vi "SC_schleife_mischer.vi"() -> ()   [LabVIEW 2019]
uses:
  Global/Global Variables/global.vi
  Global/Global Variables/Data_Display_global.vi
  Instrument_Setup.vi
  <vilib>/Analysis/NI_AALBase.lvlib
  <vilib>/Analysis/NI_AALPro.lvlib
panel:
  out "Numeric":dbl format="%#_13g"
  out "Array":dbl[](array[numeric])
  out "Numeric 5":dbl format="%#_13g"
  out "Numeric 4":dbl format="%#_13g"
  out "XY Graph 2":T1(graph)
  out "XY Graph":T1(graph)
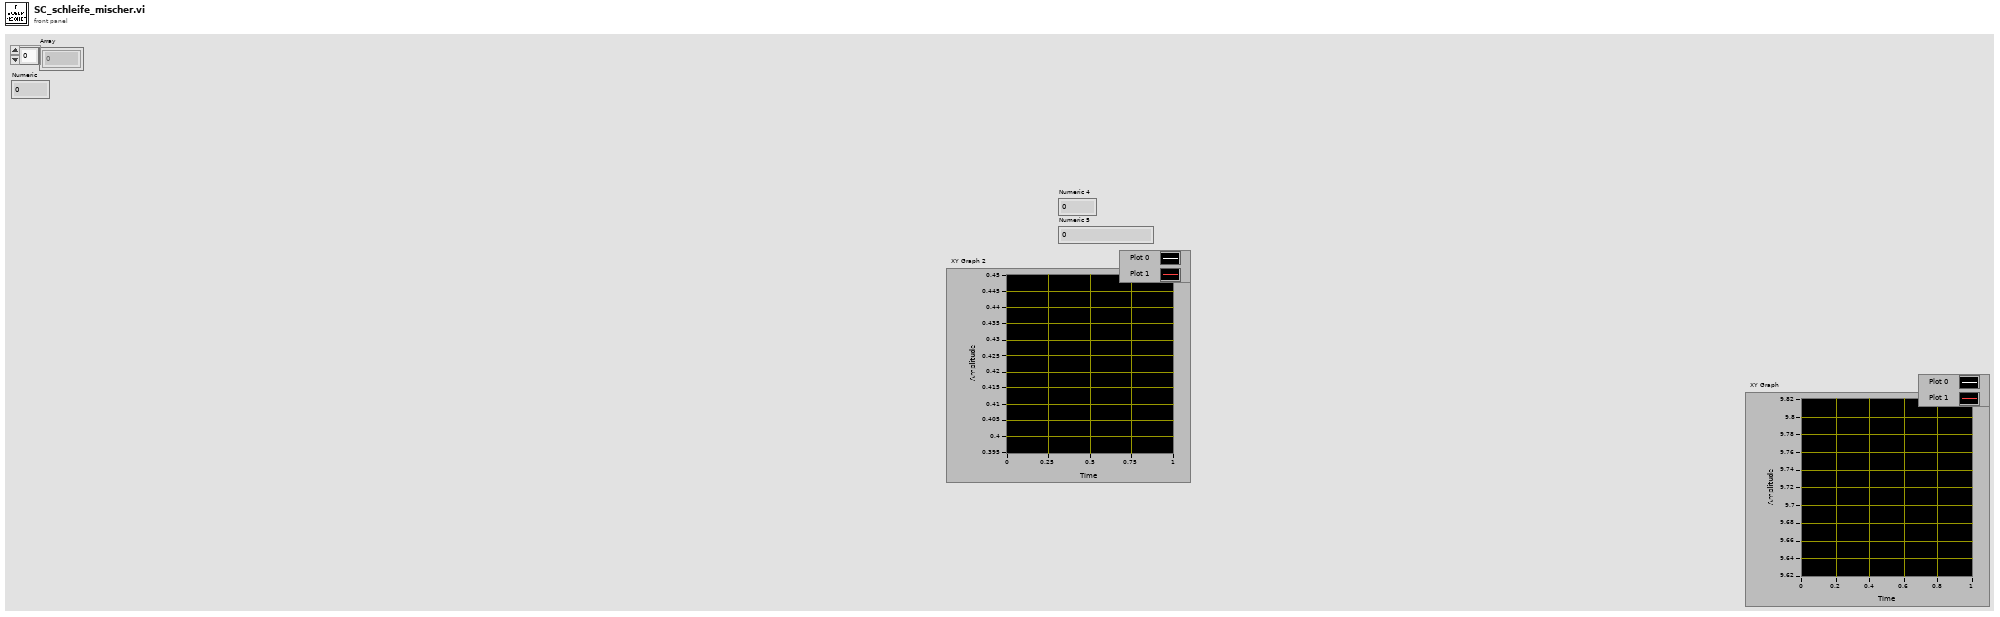
[diagram p1: front panel]
types:
  T1 = cluster{"Plot1":dbl[], "Best Linear Fit":dbl[]}[]
  T2 = typedef "LS372-Cluster.ctl" = cluster{"Activate Tsweep":bool, "Setpoint - Manual":dbl, "Rate (K/min)":dbl, "Update Lakeshores":bool, "Still Heater":bool, "Still Power (mW)":dbl, "Manual Heater":bool, "Manual Heater  (mW) ":dbl, "Heater Range":dbl, "P (Gain)":dbl, "I (Reset)":dbl, "D (Rate)":dbl, "Heater Power (mW)":dbl, "MC Thermometer":u16, "MC Temperature":dbl, "LS372-T1":dbl, "LS372 -T2":dbl, "LS372-R1 ":dbl, "LS372-R2":dbl, "LS372-T3":dbl, "LS372-T4":dbl, "LS372-R3 ":dbl, "LS372-R4 \n\n\n\n":dbl, "LS372-T5":dbl, "LS372-T6":dbl, "LS372-R5":dbl, "LS372-R6 ":dbl, "Still Power ist":dbl, "Set Temperatur Sweep main":bool, "Setpoint ist":dbl, "Disable Heater":bool}
  T3 = typedef "Ls372-Control.ctl" = cluster{"Activate Tsweep":bool, "Setpoint - Manual":dbl, "Rate (K/min)":dbl, "Update Lakeshores":bool, "Still Heater":bool, "Still Power (mW)":dbl, "Manual Heater":bool, "Manual Heater  (mW) ":dbl, "MC Thermometer":u16, "Set Temperature Sweeep main":bool, "Disable Heater":bool}
  T4 = typedef "LS350-cluster.ctl" = cluster{"Setpoint":dbl, "Heater Output":dbl, "Setpoint control":dbl, "Enable Setpoint":bool, "LS350 T1":dbl, "LS350 T2":dbl, "LS350 T3":dbl, "LS350 T4":dbl, "LS350 R1":dbl, "LS350 R2":dbl, "LS350 R3":dbl, "LS350 R4":dbl}
  T5 = cluster{"Plot 1":dbl[], "Best Linear Fit":dbl[]}[]
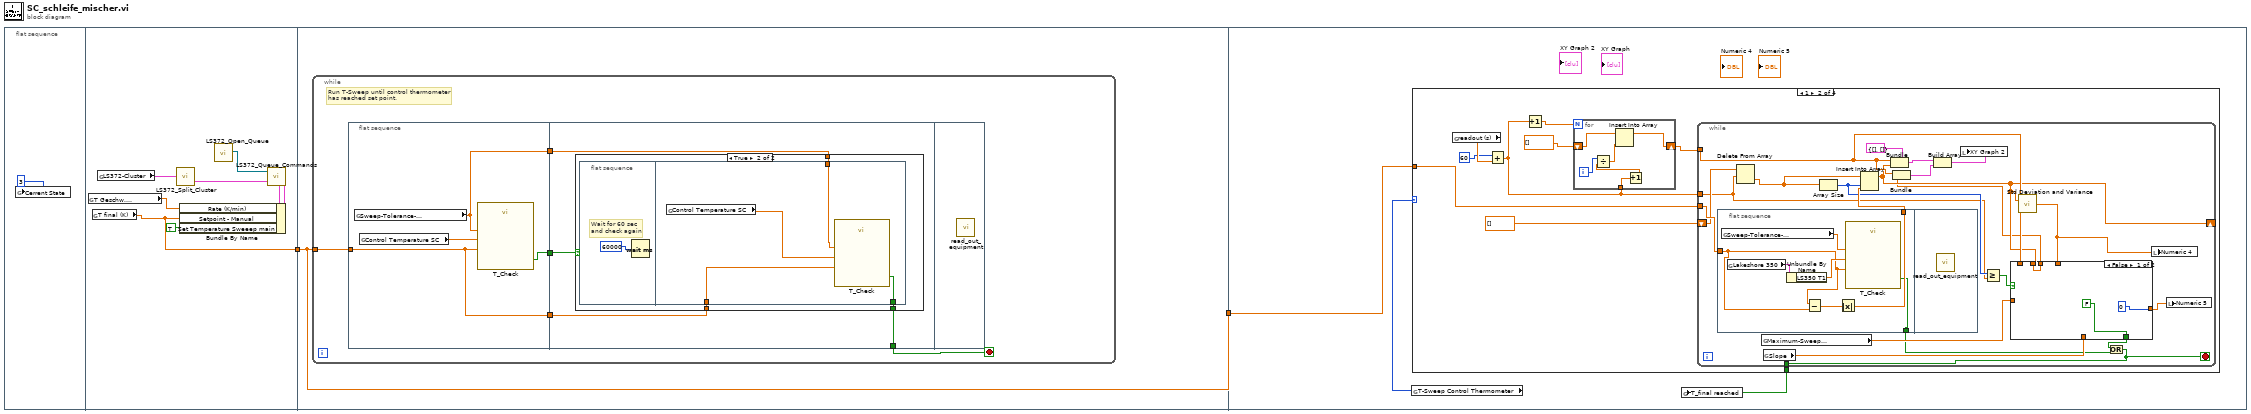
[diagram p0: block diagram]
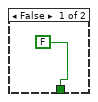
[diagram p2: hidden frame]
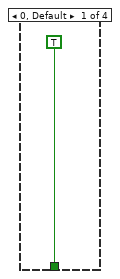
[diagram p3: hidden frame]
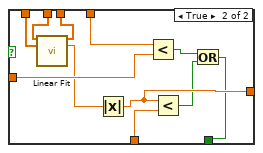
[diagram p4: hidden frame]
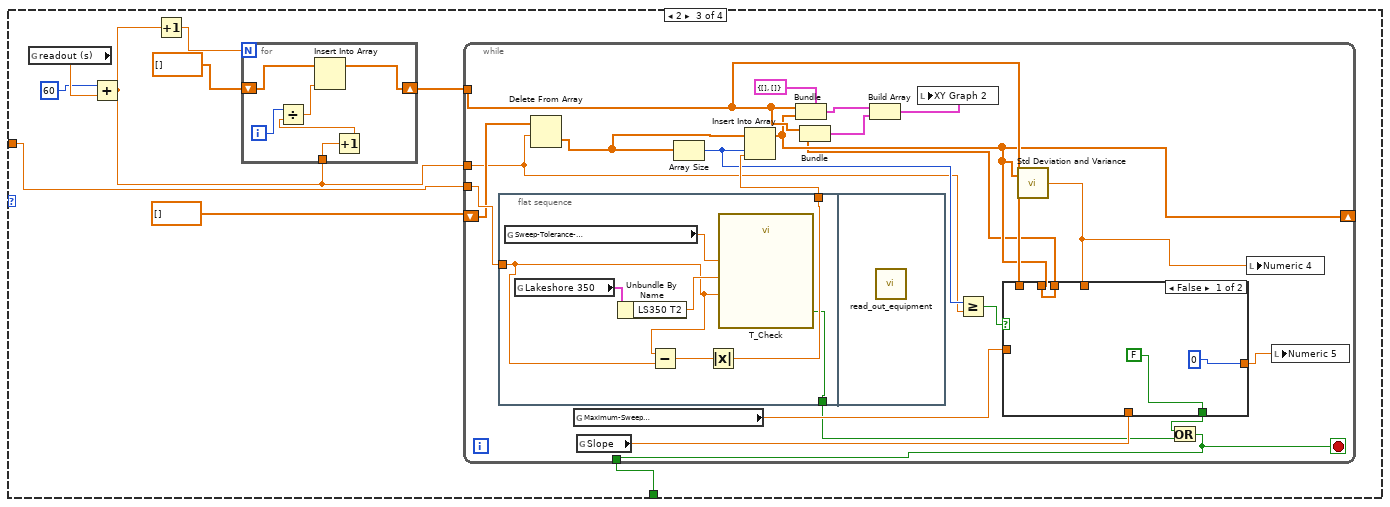
[diagram p5: hidden frame]
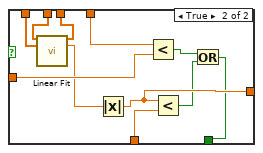
[diagram p6: hidden frame]
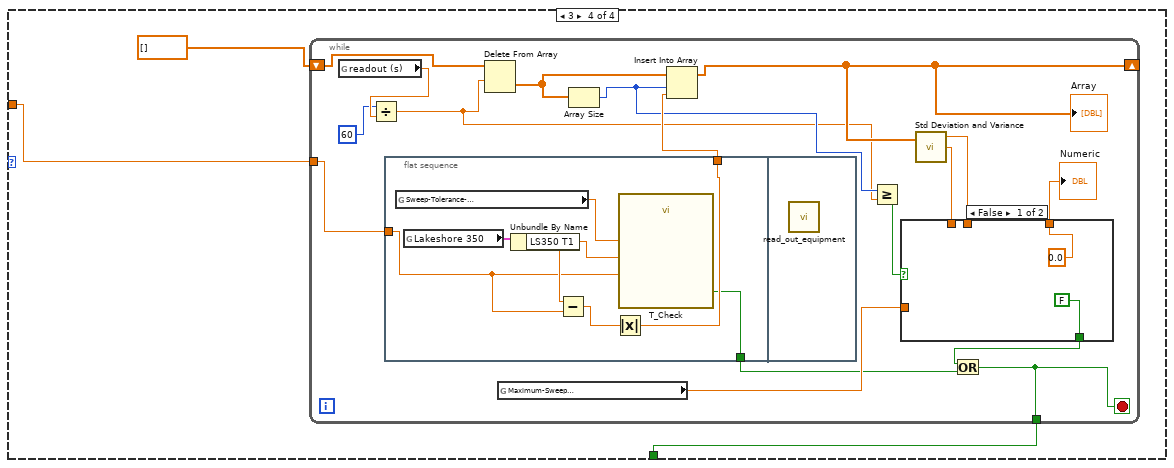
[diagram p7: hidden frame]
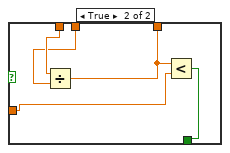
[diagram p8: hidden frame]
diagram:
  n1 = flat-sequence {
    tunnel: [w4] -> w2
    tunnel: w2 -> [w11]
    tunnel: [w11] -> w1
    tunnel: w1 -> [w35]
    frame #0 {
      n2 = global write "global.vi" "Cerrent State"(3) -> ()
    }
    frame #1 {
      n3 = global read "global.vi" "T Geschw. \n(K/min)"() -> (w7:dbl)
      n4 = global read "global.vi" "T final (K)"() -> (w4:dbl)
      n5 = global read "Data_Display_global.vi" "LS372-Cluster"() -> (w10:T2)
      n6 = call "LS372_Split_Cluster.vi"("LS372-Cluster"=w10) -> ("LS372-Control"=w9:T3)  [unwired: 1 out]
      n7 = Bundle By Name(cluster=w9, "Rate (K/min)"=w7, "Setpoint - Manual"=w4, "Set Temperature Sweeep main"=TRUE) -> (w5:T3)
      n8 = call "LS372_Open_Queue.vi"() -> ("queue out"=w6:refnum<queue>)  [unwired: 10 in, 1 out]
      n9 = call "LS372_Queue_Commands.vi"("LS372-Control"=w5, "Queue"=w6) -> ()  [unwired: 1 in, 1 out]
    }
    frame #2 {
      n10 = while {
        tunnel: w11 -> [w16]
        stop <- w12 stop-if-true
        # "Run T-Sweep until control thermometer\nhas reached set point."
        n11 = flat-sequence {
          tunnel: w16 -> [w18]
          tunnel: [w19] -> w15
          tunnel: [w18] -> w14
          tunnel: [w17] -> w13
          tunnel: w15 -> [w24]
          tunnel: w14 -> [w23]
          tunnel: w13 -> [w22]
          tunnel: [w21] -> w12
          frame #0 {
            n12 = global read "Instrument_Setup.vi" "Sweep-Tolerance-\nTemperature"() -> (w19:dbl)
            n13 = global read "Data_Display_global.vi" "Control Temperature SC"() -> (w20:dbl)
            n14 = call "T_Check.vi"("Sweep\nTolerance %"=w19, "T_target (K)"=w18, "T_in"=w20) -> ("= T target"=w17:bool)
          }
          frame #1 {
            n15 = case shown="True" w22 {
              tunnel: w23 -> [_ w28]
              tunnel: w24 -> [_ w27]
              tunnel: [FALSE w26] -> w21
              frame False {
              }
              frame True {
                n16 = flat-sequence {
                  tunnel: w28 -> [w33]
                  tunnel: w27 -> [w32]
                  tunnel: [w31] -> w26
                  frame #0 {
                    # "Wait for 60 sec\nand check again"
                    n17 = Wait (ms)(milliseconds to wait=60000) -> ()  [unwired: 1 out]
                  }
                  frame #1 {
                    n18 = global read "Data_Display_global.vi" "Control Temperature SC"() -> (w30:dbl)
                    n19 = call "T_Check.vi"("Sweep\nTolerance %"=w32, "T_target (K)"=w33, "T_in"=w30) -> ("= T target"=w31:bool)
                  }
                }
              }
            }
          }
          frame #2 {
            n20 = call "read_out_equipment.vi"() -> ()  [unwired: 1 in]
          }
        }
      }
    }
    frame #3 {
      n21 = global read "Instrument_Setup.vi" "T-Sweep Control Thermometer"() -> (w36:u16)
      n22 = case shown="1" w36 {
        tunnel: w35 -> [_ w41 w96 w154]
        tunnel: [TRUE w38 w103 w152] -> w34
        frame 0, Default {
        }
        frame 1 {
          n23 = global read "Instrument_Setup.vi" "readout (s)"() -> (w46:dbl)
          n24 = Add(x=60, y=w46) -> (x+y=w39:dbl)
          n25 = Increment(x=w39) -> (x+1=w44:dbl)
          n26 = for {
            N: w44 -> [_]
            shift-right: [w91] -> w40
            shift-left: dbl[] [] -> [w93]
            tunnel: w39 -> [w90]
            i -> [w94]
            n27 = Increment(x=w90) -> (x+1=w89:dbl)
            n28 = Divide(x=w94, y=w89) -> (x/y=w92:dbl)
            n29 = Insert Into Array(array=w93, new element=w92) -> (w91:dbl[])  [unwired: 1 in]
          }
          n30 = while {
            shift-right: [w56] -> _
            shift-left: dbl[] [] -> [w66]
            tunnel: w41 -> [w67]
            tunnel: w40 -> [w59]
            tunnel: w39 -> [w57]
            tunnel: [w47] -> w38
            stop <- w47 stop-if-true
            n31 = flat-sequence {
              tunnel: w67 -> [w85]
              tunnel: [w83] -> w63
              tunnel: [w82] -> w49
              frame #0 {
                n32 = global read "Instrument_Setup.vi" "Sweep-Tolerance-\nTemperature"() -> (w88:dbl)
                n33 = global read "Data_Display_global.vi" "Lakeshore 350"() -> (w87:T4)
                n34 = Unbundle By Name(w87) -> ("LS350 T1"=w86:dbl)
                n35 = Subtract(x=w85, y=w85) -> (x-y=w84:dbl)
                n36 = Absolute Value(x=w84) -> (abs(x)=w83:dbl)
                n37 = call "T_Check.vi"("Sweep\nTolerance %"=w88, "T_target (K)"=w85, "T_in"=w86) -> ("= T target"=w82:bool)
              }
              frame #1 {
                n38 = call "read_out_equipment.vi"() -> ()  [unwired: 1 in]
              }
            }
            n39 = Delete From Array(array=w66, length=w57) -> (deleted portion=w64:dbl[])  [unwired: 1 in, 1 out]
            n40 = global read "Instrument_Setup.vi" "Maximum-Sweep\nSettle %/min"() -> (w52:dbl)
            n41 = global read "Instrument_Setup.vi" "Slope"() -> (w51:dbl)
            n42 = Array Size(array=w64) -> (size(s)=w58:i32)
            n43 = Insert Into Array(array=w64, index=w58, new element=w63) -> (w56:dbl[])
            n44 = Bundle(cluster=cluster{"Plot 1":dbl[], "Plot 2":dbl[]} {"Plot 1"=[], "Plot 2"=[]}, "Plot 1"=w59, "Plot 2"=w56) -> (w62:cluster{"Plot 1":dbl[], "Plot 2":dbl[]})
            n45 = Greater Or Equal?(x=w58, y=w57) -> (x >= y?=w53:bool)
            n46 = call <vilib>:"Std Deviation and Variance.vi"("X"=w56) -> ("standard deviation"=w55:dbl)  [unwired: 1 in, 2 out]
            n47 = case shown="False" w53 {
              tunnel: w56 -> [w68 w80]
              tunnel: w59 -> [_ w81]
              tunnel: w55 -> [_ w78]
              tunnel: [w68 w79] -> w54
              tunnel: w52 -> [_ w77]
              tunnel: w51 -> [_ w75]
              tunnel: [0 w74] -> w50
              tunnel: [FALSE w71] -> w48
              frame False {
              }
              frame True {
                n48 = call <vilib>:"Linear Fit.vi"("Y"=w80, "X"=w81) -> ("Best Linear Fit"=w79:dbl[], "slope"=w76:dbl)  [unwired: 9 in, 3 out]
                n49 = Absolute Value(x=w76) -> (abs(x)=w74:dbl)
                n50 = Less?(x=w78, y=w77) -> (x < y?=w73:bool)
                n51 = Less?(x=w74, y=w75) -> (x < y?=w72:bool)
                n52 = Or(x=w73, y=w72) -> (x .or. y?=w71:bool)
              }
            }
            n53 = Bundle(w59, "Best Linear Fit"=w54) -> (w61:cluster{dbl[], "Best Linear Fit":dbl[]})  [unwired: 1 in]
            n54 = Build Array(w62, w61) -> (w60:T5)
            n55 = local write "XY Graph 2"(w60) -> ()
            n56 = Or(x=w48, y=w49) -> (x .or. y?=w47:bool)
            n57 = local write "Numeric 4"(w55) -> ()
            n58 = local write "Numeric 5"(w50) -> ()
          }
        }
        frame 2 {
          n59 = global read "Instrument_Setup.vi" "readout (s)"() -> (w102:dbl)
          n60 = Add(x=60, y=w102) -> (x+y=w97:dbl)
          n61 = Increment(x=w97) -> (x+1=w100:dbl)
          n62 = for {
            N: w100 -> [_]
            shift-right: [w106] -> w98
            shift-left: dbl[] [] -> [w108]
            tunnel: w97 -> [w105]
            i -> [w109]
            n63 = Increment(x=w105) -> (x+1=w104:dbl)
            n64 = Divide(x=w109, y=w104) -> (x/y=w107:dbl)
            n65 = Insert Into Array(array=w108, new element=w107) -> (w106:dbl[])  [unwired: 1 in]
          }
          n66 = while {
            shift-right: [w119] -> _
            shift-left: dbl[] [] -> [w129]
            tunnel: w96 -> [w130]
            tunnel: w98 -> [w122]
            tunnel: w97 -> [w120]
            tunnel: [w110] -> w103
            stop <- w110 stop-if-true
            n67 = flat-sequence {
              tunnel: w130 -> [w148]
              tunnel: [w146] -> w126
              tunnel: [w145] -> w112
              frame #0 {
                n68 = global read "Instrument_Setup.vi" "Sweep-Tolerance-\nTemperature"() -> (w151:dbl)
                n69 = global read "Data_Display_global.vi" "Lakeshore 350"() -> (w150:T4)
                n70 = Unbundle By Name(w150) -> ("LS350 T2"=w149:dbl)
                n71 = Subtract(x=w148, y=w148) -> (x-y=w147:dbl)
                n72 = Absolute Value(x=w147) -> (abs(x)=w146:dbl)
                n73 = call "T_Check.vi"("Sweep\nTolerance %"=w151, "T_target (K)"=w148, "T_in"=w149) -> ("= T target"=w145:bool)
              }
              frame #1 {
                n74 = call "read_out_equipment.vi"() -> ()  [unwired: 1 in]
              }
            }
            n75 = Delete From Array(array=w129, length=w120) -> (deleted portion=w127:dbl[])  [unwired: 1 in, 1 out]
            n76 = global read "Instrument_Setup.vi" "Maximum-Sweep\nSettle %/min"() -> (w115:dbl)
            n77 = global read "Instrument_Setup.vi" "Slope"() -> (w114:dbl)
            n78 = Array Size(array=w127) -> (size(s)=w121:i32)
            n79 = Insert Into Array(array=w127, index=w121, new element=w126) -> (w119:dbl[])
            n80 = Bundle(cluster=cluster{"Plot 1":dbl[], "Plot 2":dbl[]} {"Plot 1"=[], "Plot 2"=[]}, "Plot 1"=w122, "Plot 2"=w119) -> (w125:cluster{"Plot 1":dbl[], "Plot 2":dbl[]})
            n81 = Greater Or Equal?(x=w121, y=w120) -> (x >= y?=w116:bool)
            n82 = call <vilib>:"Std Deviation and Variance.vi"("X"=w119) -> ("standard deviation"=w118:dbl)  [unwired: 1 in, 2 out]
            n83 = case shown="False" w116 {
              tunnel: w119 -> [w131 w143]
              tunnel: w122 -> [_ w144]
              tunnel: w118 -> [_ w141]
              tunnel: [w131 w142] -> w117
              tunnel: w115 -> [_ w140]
              tunnel: w114 -> [_ w138]
              tunnel: [0 w137] -> w113
              tunnel: [FALSE w134] -> w111
              frame False {
              }
              frame True {
                n84 = call <vilib>:"Linear Fit.vi"("Y"=w143, "X"=w144) -> ("Best Linear Fit"=w142:dbl[], "slope"=w139:dbl)  [unwired: 9 in, 3 out]
                n85 = Absolute Value(x=w139) -> (abs(x)=w137:dbl)
                n86 = Less?(x=w141, y=w140) -> (x < y?=w136:bool)
                n87 = Less?(x=w137, y=w138) -> (x < y?=w135:bool)
                n88 = Or(x=w136, y=w135) -> (x .or. y?=w134:bool)
              }
            }
            n89 = Bundle(w122, "Best Linear Fit"=w117) -> (w124:cluster{dbl[], "Best Linear Fit":dbl[]})  [unwired: 1 in]
            n90 = Build Array(w125, w124) -> (w123:T5)
            n91 = local write "XY Graph 2"(w123) -> ()
            n92 = Or(x=w111, y=w112) -> (x .or. y?=w110:bool)
            n93 = local write "Numeric 4"(w118) -> ()
            n94 = local write "Numeric 5"(w113) -> ()
          }
        }
        frame 3 {
          n95 = while {
            tunnel: w154 -> [w167]
            shift-right: [w165] -> _
            shift-left: dbl[] [] -> [w169]
            tunnel: [w155] -> w152
            stop <- w155 stop-if-true
            n96 = global read "Instrument_Setup.vi" "readout (s)"() -> (w171:dbl)
            n97 = Divide(x=60, y=w171) -> (x/y=w160:dbl)
            n98 = flat-sequence {
              tunnel: w167 -> [w182]
              tunnel: [w180] -> w166
              tunnel: [w179] -> w156
              frame #0 {
                n99 = global read "Instrument_Setup.vi" "Sweep-Tolerance-\nTemperature"() -> (w185:dbl)
                n100 = global read "Data_Display_global.vi" "Lakeshore 350"() -> (w184:T4)
                n101 = Unbundle By Name(w184) -> ("LS350 T1"=w183:dbl)
                n102 = Subtract(x=w183, y=w182) -> (x-y=w181:dbl)
                n103 = Absolute Value(x=w181) -> (abs(x)=w180:dbl)
                n104 = call "T_Check.vi"("Sweep\nTolerance %"=w185, "T_target (K)"=w182, "T_in"=w183) -> ("= T target"=w179:bool)
              }
              frame #1 {
                n105 = call "read_out_equipment.vi"() -> ()  [unwired: 1 in]
              }
            }
            n106 = Delete From Array(array=w169, length=w160) -> (deleted portion=w168:dbl[])  [unwired: 1 in, 1 out]
            n107 = global read "Instrument_Setup.vi" "Maximum-Sweep\nSettle %/min"() -> (w158:dbl)
            n108 = Array Size(array=w168) -> (size(s)=w161:i32)
            n109 = Insert Into Array(array=w168, index=w161, new element=w166) -> (w165:dbl[])
            "Array" <- w165
            n110 = Greater Or Equal?(x=w161, y=w160) -> (x >= y?=w159:bool)
            n111 = call <vilib>:"Std Deviation and Variance.vi"("X"=w165) -> ("mean"=w164:dbl, "standard deviation"=w163:dbl)  [unwired: 1 in, 1 out]
            n112 = case shown="False" w159 {
              tunnel: w164 -> [_ w177]
              tunnel: w163 -> [_ w178]
              tunnel: [0.0 w176] -> w162
              tunnel: w158 -> [_ w175]
              tunnel: [FALSE w174] -> w157
              frame False {
              }
              frame True {
                n113 = Divide(x=w178, y=w177) -> (x/y=w176:dbl)
                n114 = Less?(x=w176, y=w175) -> (x < y?=w174:bool)
              }
            }
            "Numeric" <- w162
            n115 = Or(x=w157, y=w156) -> (x .or. y?=w155:bool)
          }
        }
      }
      n116 = global write "Data_Display_global.vi" "T_final reached"(w34) -> ()
    }
  }
